vi "IMIC_SetDevice.vi"(2 "Value":dbl, 3 "DeviceID":i32(ring) items=["EndLoop"=-2, "Loop"=-1, "Invalid"=0, "TriggerPolyV"=1, "TriggerCamera"=2, "SyncCamera"=3, "Do1"=1000, "Do2"=1001, "Do3"=1002, "Do4"=1003, "Do5"=1004, "Do6"=1005, "Do7"=1006, "Do8"=1007, "Do9"=1008, "Do10"=1009, "Do11"=1010, "Do12"=1011, "Do13"=1012, "Do14"=1013, "Do15"=1014, "Do16"=1015, "Do17"=1016, "Do18"=1017, "Do19"=1018, "Do20"=1019, "Do21"=1020, "Do22"=1021, "Do23"=1022, "Do24"=1023, "Do_End"=1024, "Da1"=2000, "Da2"=2001, "Da3"=2002, "Da4"=2003, "Da5"=2004, "Da6"=2005, "Da7"=2006, "Da8"=2007, "DaIncr_First"=2008, "Da1Incr"=2100, "Da2Incr"=2101, "Da3Incr"=2102, "Da4Incr"=2103, "Da5Incr"=2104, "Da6Incr"=2105, "Da7Incr"=2106, "Da8Incr"=2107, "Da1Raw"=2200, "Da2Raw"=2201, "Da3Raw"=2202, "Da4Raw"=2203, "Da5Raw"=2204, "Da6Raw"=2205, "Da7Raw"=2206, "Da8Raw"=2207, "Da1RawIncr"=2300, "Da2RawIncr"=2301, "Da3RawIncr"=2302, "Da4RawIncr"=2303, "Da5RawIncr"=2304, "Da6RawIncr"=2305, "Da7RawIncr"=2306, "Da8RawIncr"=2307, "Uart1"=3000, "Uart2"=3001, "Uart3"=3002, "Uart_End"=3003, "Di1"=4000, "Di2"=4001, "Di3"=4002, "Di4"=4003, "Di5"=4004, "Di6"=4005, "Di7"=4006, "Di8"=4007, "Di9"=4008, "Di10"=4009, "Di11"=4010, "Di12"=4011, "Di13"=4012, "Di14"=4013, "Di15"=4014, "Di16"=4015, "Di17"=4016, "Di18"=4017, "Di19"=4018, "Di20"=4019, "Di21"=4020, "Di22"=4021, "Di23"=4022, "Di24"=4023, "Di_End"=4024, "ICU_End"=4025, "LedIllum"=10000, "ImicAxisXRel"=11000, "ImicAxisYRel"=11001, "ImicAxisZRel"=11002, "ImicAxisTurretRel"=11003, "ImicAxisFilter1Rel"=11004, "ImicAxisFilter2Rel"=11005, "ImicAxis_End"=11006, "ImicAxisXAbs"=11200, "ImicAxisYAbs"=11201, "ImicAxisZAbs"=11202, "ImicAxisTurretAbs"=11203, "ImicAxisFilter1Abs"=11204, "ImicAxisFilter2Abs"=11205, "ImicAxisXVel"=11300, "ImicAxisYVel"=11301, "ImicAxisZVel"=11302, "ImicAxisTurretVel"=11303, "ImicAxisFilter1Vel"=11304, "ImicAxisFilter2Vel"=11305, "ImicAxisXMoving"=11400, "ImicAxisYMoving"=11401, "ImicAxisZMoving"=11402, "ImicAxisTurretMoving"=11403, "ImicAxisFilter1Moving"=11404, "ImicAxisFilter2Moving"=11405, "ImicPiezoClip"=12001, "ImicPiezo"=12002, "IMIC_End"=12003], 4 "handle":u64) -> (0 "handle out":u64, 1 "output param":T1(ring))   [LabVIEW 2011]
uses:
  tillimic32.dll
panel:
  # "dll version 21: geht noch nicht viel\nv27: xrel,yrel,zrel:OK, units mm\n     filter1,2abs:OK, unist 0,1,2\n     Turret:Nein\n     Piezo:Nein,Da4raw:Nein, aber Da4 0..10V: OK\n\nNon reentrant?!"
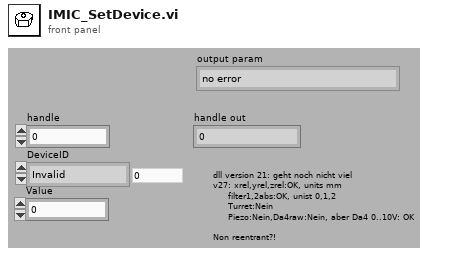
[diagram p1: front panel]
types:
  T1 = enum16{"no error", "missing axis", "missing Z axis", "missing Filter", "iMic not initialized", "no property", "wrong handle", "protocol not finished", "user parameter to long (>32 bits)", "no user parameter handle", "failed to open comport", "failed to initialize"}
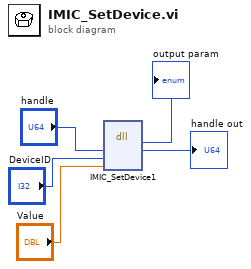
[diagram p0: block diagram]
diagram:
  n1 = dll-call lib="D:/Colibri/Drivers/TILLPhotonics/tillimic*.*" fn="IMIC_SetDevice1"("handle"="handle", "DevID"="DeviceID", "Value"="Value") -> ("return type"=→"output param":i32, "handle"=→"handle out":u64)  [unwired: 5 in, 2 out]
